vi "HB_CloseHuskieBoard.vi"(8 "error in (no error)":errorcluster, 11 "HBDeviceRef":T1) -> (0 "error out":errorcluster)   [LabVIEW 2016]
doc: "Closes the serial connection between the roboRIO and the Huskie Board."
uses:
  <vilib>/Rock Robotics/WPI/SerialPort/WPI_SerialPortRef.ctl
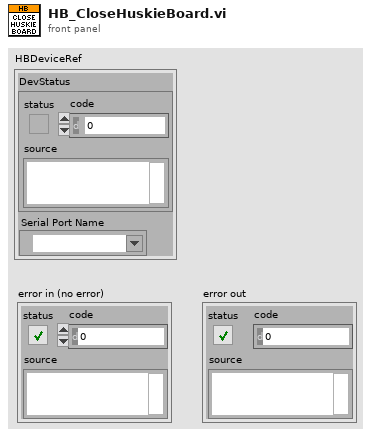
[diagram p1: front panel]
types:
  T1 = typedef "WPI_SerialPortRef.ctl" = cluster{"DevStatus":errorcluster, "Serial Port Name":refnum<visa-resource-name>}
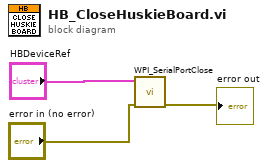
[diagram p0: block diagram]
diagram:
  n1 = call <vilib>:"WPI_SerialPortClose.vi"("error in (no error)"="error in (no error)", "SerialPortRef"="HBDeviceRef") -> ("error out"=→"error out":errorcluster)  [unwired: 9 in]
